vi "SFTP List Directory.vi"() -> ()   [LabVIEW 2023]
doc: "<b>This example, while not specifically written for the LabVIEW Real-Time Module, runs on RT targets.</b>\n\nDemonstrates listing the directory contents of an SFTP server."
uses:
  <vilib>/net/SFTP/File Attributes/File Attributes.lvclass/File Attributes.ctl
  <vilib>/net/SFTP/File Attributes/Read filename.vi
  <vilib>/net/SFTP/File Attributes/Read longname.vi
  <vilib>/net/SFTP/File Attributes/Report item not found.vi
  <vilib>/net/SFTP/Connect (OpenSSH).vi
  <vilib>/Utility/error.llb/Error Cluster From Error Code.vi
  <vilib>/net/SFTP/Session/Session.lvclass
  <vilib>/net/SFTP/NI_SFTP.lvlib
  <vilib>/net/SFTP/File Attributes/File Attributes.lvclass
panel:
  out "Directory Contents":T1(array[cluster])
  in  "Directory":string="."
  in  "user@host":string
  # "Overview: Demonstrates using the SFTP VIs to log into a remote SFTP server and view the contents of a directory.\nInstructions:\n1. This example assumes that all authentication is automatic and has already been configured.\n2. This example defaults to connecting via OpenSSH (`ssh`; `sftp`). If you wish to connect via PuTTY (`plink`, `psftp`), open the block diagram and adjust the SFTP Connect instance.\n3. Open an operating system command prompt and confirm that you can login to the remote server without a password. For instance, if you are using PuTTY to connect to an NI Linux RT system at address 1.2.3.4, you should see precisely the following at the command prompt:\n\n>psftp admin@1.2.3.4\nUsing username \"admin\".\nPre-authentication banner message from server:\n| NI Linux Real-Time (run mode)\n|\n| Log in with your NI-Auth credentials.\n|\nEnd of banner message from server\nRemote working directory is /home/admin\npsftp>\n\n4. Set user@host. Set Directory if desired.\n5. Run the VI. \n6. Directory Contents lists the files in the specified directory. Both the filename itself and its \"long listing\" are displayed. The long listing is a textual representation of the file metadata similar to the output of the FTP \"dir\" command or the Unix \"ls -l\" command."
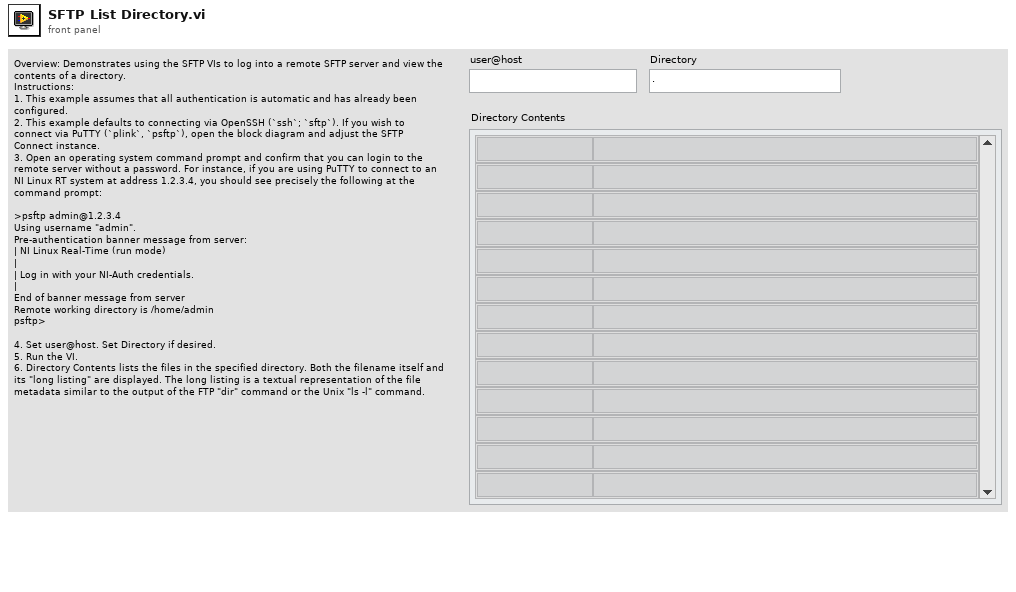
[diagram p1: front panel]
types:
  T1 = cluster{"filename":string, "long listing":string}[]
  T2 = cluster{"Properties:Name":string, "Properties:Long Listing":string}
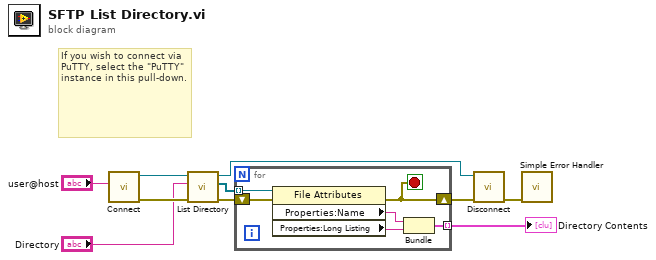
[diagram p0: block diagram]
diagram:
  # "If you wish to connect via PuTTY, select the \"PuTTY\" instance in this pull-down."
  n1 = call-poly <vilib>:"Connect.vi"("user@host"="user@host") -> ("error out"=w9:errorcluster, "session"=w10:refnum<class "Session.lvclass">)  [unwired: 9 in]
  n2 = call <vilib>:"List Directory.vi"("error in (no error)"=w9, "remote path"="Directory", "session in"=w10) -> ("error out"=w6:errorcluster, "files and directories"=w7:refnum<class "File Attributes.lvclass">[], "session out"=w8:refnum<class "Session.lvclass">)  [unwired: 6 in]
  n3 = for {
    tunnel: w7 -> [w16] mode=indexing
    tunnel: [w12] -> w2 mode=indexing
    shift-right: [w11] -> w1
    shift-left: w6 -> [w15]
    stop <- w11 stop-if-true
    n4 = property class="File Attributes"(reference=w16, error in=w15) -> (error out=w11:errorcluster, "Properties:Name"=w13:string, "Properties:Long Listing"=w14:string)  [unwired: 1 out]
    n5 = Bundle("Properties:Name"=w13, "Properties:Long Listing"=w14) -> (w12:T2)  [unwired: 1 in]
  }
  "Directory Contents" <- w2
  n6 = call-dynamic "Disconnect.vi"("error in"=w1, "session in"=w8) -> ("error out"=w5:errorcluster)  [unwired: 6 in, 3 out]
  n7 = call <vilib>:"Simple Error Handler.vi"("error in (no error)"=w5) -> ()  [unwired: 4 in, 5 out]
